vi "计算结果-步响应.vi"(5 "油动机试验路径":path=path "D:/研究生/课程/油动机项目/实验文件夹/DR96-03-5/GV1") -> (0 "步响应计算参数 out":T2, 2 "波形图":cluster{dbl, dbl, dbl[][]}(graph))   [LabVIEW 2013]
uses:
  <vilib>/Analysis/3filter.llb/Filter Passband Type.ctl
  <vilib>/Analysis/3filter.llb/Butterworth Filter (DBL).vi
  <vilib>/Analysis/NI_AALBase.lvlib
panel:
  out "波形图 2":dbl[](graph) caption="波形图"
  in  "步响应控制参数":T1={"rise_step"=1.0, "rise_criterion"=200.0, "peak_step"=1.0, "peak_criterion"=40.0, "nb_of_peaks"=200.0}
  in  "步响应计算参数 in":T2
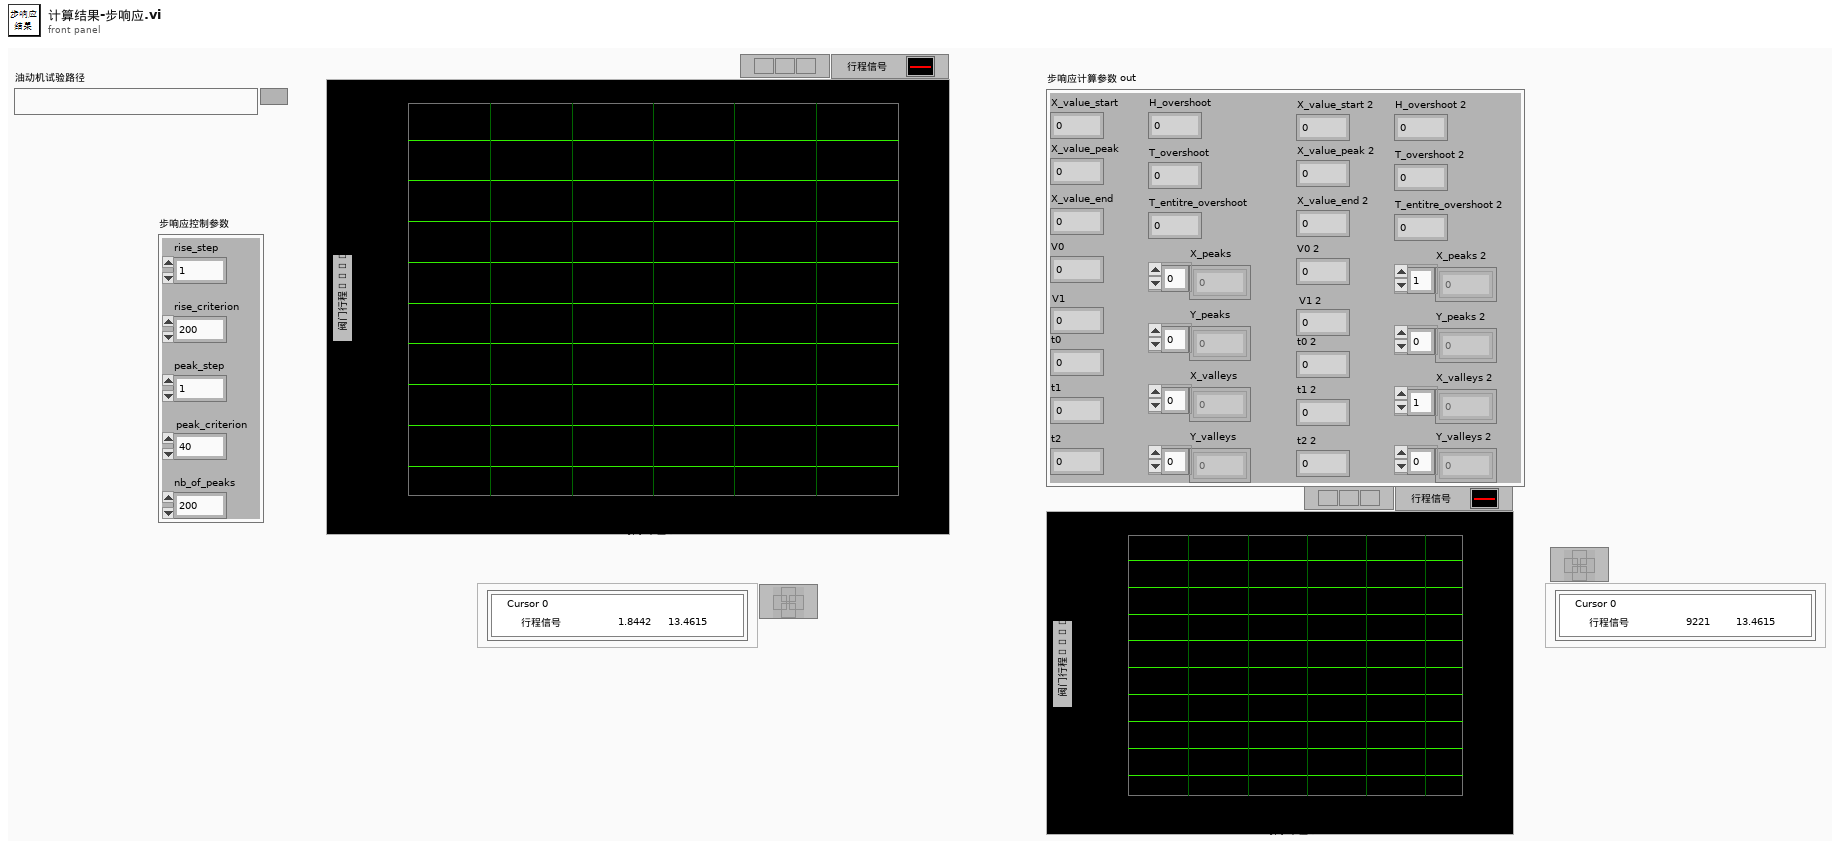
[diagram p1: front panel]
types:
  T1 = cluster{"rise_step":dbl, "rise_criterion":dbl, "peak_step":dbl, "peak_criterion":dbl, "nb_of_peaks":dbl}
  T2 = cluster{"X_value_start":dbl, "X_value_peak":dbl, "t1":dbl, "X_value_end":dbl, "V0":dbl, "V1":dbl, "t0":dbl, "X_peaks":dbl[], "X_valleys":dbl[], "Y_peaks":dbl[], "Y_valleys":dbl[], "t2":dbl, "H_overshoot":dbl, "T_overshoot":dbl, "T_entitre_overshoot":dbl, "X_value_start 2":dbl, "X_value_peak 2":dbl, "t1 2":dbl, "X_value_end 2":dbl, "V0 2":dbl, "V1 2":dbl, "t0 2":dbl, "X_peaks 2":dbl[], "X_valleys 2":dbl[], "Y_peaks 2":dbl[], "t2 2":dbl, "H_overshoot 2":dbl, "T_overshoot 2":dbl, "T_entitre_overshoot 2":dbl, "Y_valleys 2":dbl[]}
  T3 = typedef "NI_AALBase.lvlib/Filter Passband Type.ctl" = enum32{"Lowpass", "Highpass", "Bandpass", "Bandstop"}
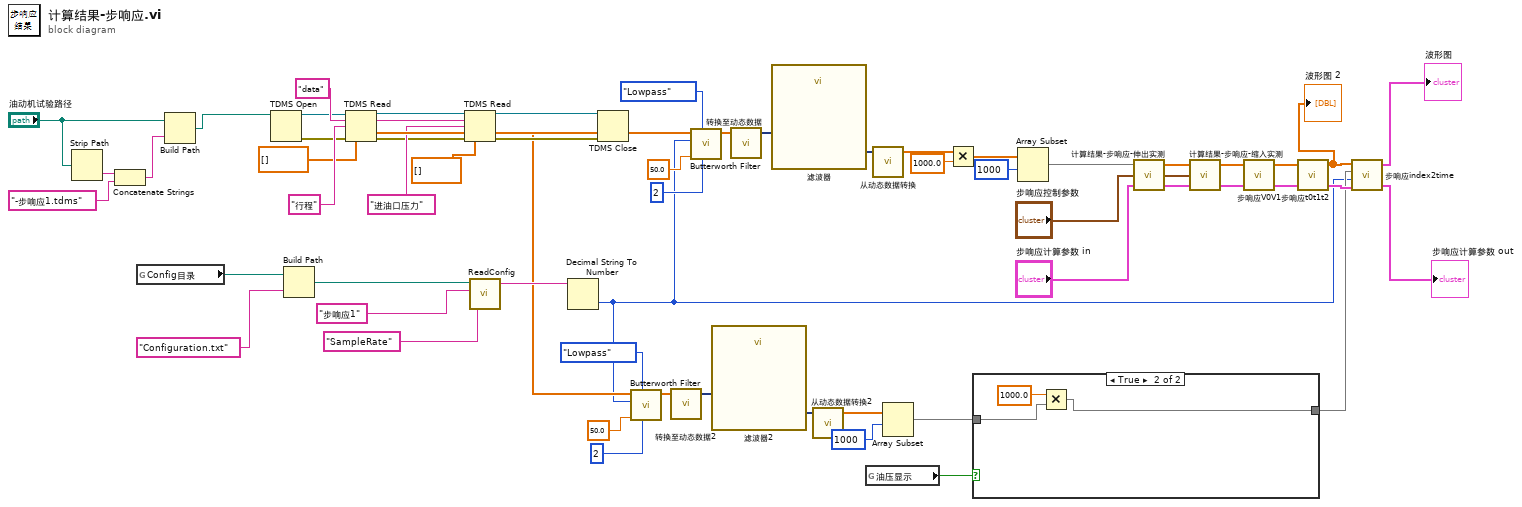
[diagram p0: block diagram]
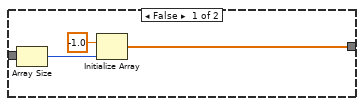
[diagram p2: hidden frame]
diagram:
  n1 = Strip Path(path="油动机试验路径") -> (name=w45:string)  [unwired: 1 out]
  n2 = Concatenate Strings(w45, "-步响应1.tdms") -> (w43:string)
  n3 = global read "Config目录.vi" "Config目录"() -> (w23:path)
  n4 = Build Path(base path="油动机试验路径", name or relative path=w43) -> (appended path=w42:path)
  n5 = TDMS Open(11:w42) -> (0:w47:errorcluster, 3:w46:refnum<k34>)  [unwired: 6 in]
  n6 = Build Path(base path=w23, name or relative path="Configuration.txt") -> (appended path=w22:path)
  n7 = TDMS Read(0:w46, 5:"data" ("组名称输入"), 7:"行程" ("通道名输入"), 11:w47, 12:dbl[] []) -> (4:w16:refnum<k34>, 6:w15:string, 10:w55:dbl[], 15:w18:errorcluster)  [unwired: 3 in, 2 out]
  n8 = TDMS Read(0:w16, 5:w15, 7:"进油口压力" ("组名称输入"), 11:w18, 12:dbl[] []) -> (4:w17:refnum<k34>, 10:w3:dbl[], 15:w19:errorcluster)  [unwired: 3 in, 3 out]
  n9 = call "ReadConfig.vi"("Key"="SampleRate", "Section"="步响应1", "Path"=w22) -> ("Value"=w27:string)  [unwired: 1 in, 2 out]
  n10 = Decimal String To Number(string=w27) -> (number=w2:i32)  [unwired: 2 in, 1 out]
  n11 = TDMS Close(8:w19, 11:w17) -> ()  [unwired: 2 out]
  n12 = call-poly <vilib>:"Butterworth Filter.vi"("order"=2, "filter type"=Filter_Passband_Type."Lowpass", "low cutoff freq: fl"=50.0, "sampling freq: fs"=w2, "X"=w3) -> ("Filtered X"=w8:dbl[])  [unwired: 3 in, 1 out]
  n13 = call "转换至动态数据2"("Array"=w8) -> ("Dynamic Data Type"=w9:dynamicdata)  [unwired: 3 in]
  n14 = call-poly <vilib>:"Butterworth Filter.vi"("order"=2, "filter type"=Filter_Passband_Type."Lowpass", "low cutoff freq: fl"=50.0, "sampling freq: fs"=w2, "X"=w55) -> ("Filtered X"=w52:dbl[])  [unwired: 3 in, 1 out]
  n15 = call "滤波器2"("Signal"=w9) -> ("Filtered Signal"=w10:dynamicdata)  [unwired: 9 in, 1 out]
  n16 = call "转换至动态数据"("Array"=w52) -> ("Dynamic Data Type"=w53:dynamicdata)  [unwired: 3 in]
  n17 = call "滤波器"("Signal"=w53) -> ("Filtered Signal"=w54:dynamicdata)  [unwired: 9 in, 1 out]
  n18 = call "从动态数据转换2"("Dynamic Data Type"=w10) -> ("Array"=w4:dbl[])  [unwired: 3 in]
  n19 = global read "油压显示.vi" "油压显示"() -> (w13:bool)
  n20 = call "从动态数据转换"("Dynamic Data Type"=w54) -> ("Array"=w57:dbl[])  [unwired: 3 in]
  n21 = Array Subset(array=w4, index=1000) -> (w12:dbl[])  [unwired: 1 in]
  n22 = Multiply(x=w57, y=1000.0) -> (x*y=w61:dbl[])
  n23 = case shown="True" w13 {
    tunnel: w12 -> [w65 w67]
    tunnel: [w62 w66] -> w11
    frame False {
      n24 = Array Size(array=w65) -> (size(s)=w64:i32)
      n25 = Initialize Array(-1.0 ("element"), w64) -> (w62:dbl[])
    }
    frame True {
      n26 = Multiply(x=1000.0 ("low cutoff freq: fl"), y=w67) -> (x*y=w66:dbl[])
    }
  }
  n27 = Array Subset(array=w61, index=1000 ("索引")) -> (w40:dbl[])  [unwired: 1 in]
  n28 = call "计算结果-步响应-伸出实测.vi"("步响应计算参数 in"="步响应计算参数 in", "步响应控制参数 in"="步响应控制参数", "行程 in"=w40) -> ("步响应计算参数 out"=w38:T2, "步响应控制参数 out"=w28:T1, "行程 out"=w29:dbl[])
  n29 = call "计算结果-步响应-缩入实测.vi"("步响应计算参数 in"=w38, "步响应控制参数"=w28, "行程 in"=w29) -> ("步响应计算参数 out"=w33:T2, "行程 out"=w34:dbl[])  [unwired: 1 in]
  n30 = call "步响应V0V1.vi"("步响应计算参数 in"=w33, "行程 in"=w34) -> ("步响应计算参数 out"=w37:T2, "行程 out"=w36:dbl[])  [unwired: 2 in]
  n31 = call "步响应t0t1t2.vi"("步响应计算参数 in"=w37, "行程 in"=w36) -> ("步响应计算参数 out"=w35:T2, "行程 out"=w1:dbl[])  [unwired: 2 in]
  "波形图 2" <- w1
  n32 = call "步响应index2time.vi"("步响应计算参数 in"=w35, "Sampling Rate"=w2, "油压1"=w11, "行程 in"=w1) -> ("步响应计算参数 out"=→"步响应计算参数 out":T2, "Waveform Graph"=→"波形图":cluster{dbl, dbl, dbl[][]})  [unwired: 1 in]
